vi "get response.vi"(8 "error in (no error)":errorcluster, 9 "time out (ms)":u32=30000, 10 "end char":string="^", 11 "port number":refnum<visa-resource-name>) -> (0 "error out":errorcluster, 1 "timed out":bool, 2 "response":string, 3 "port number out":refnum<visa-resource-name>)   [LabVIEW 2012]
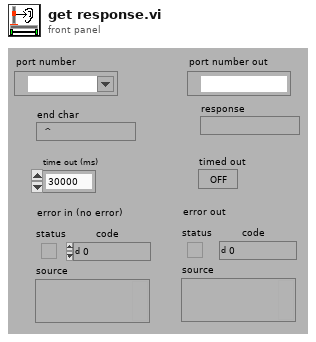
[diagram p1: front panel]
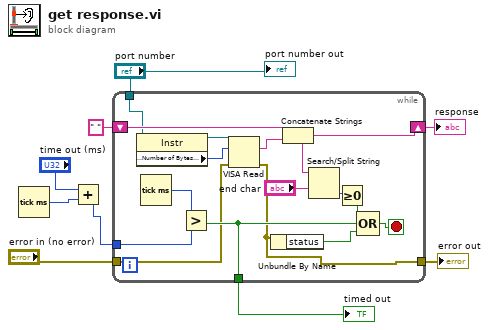
[diagram p0: block diagram]
diagram:
  n1 = Tick Count (ms)() -> (millisecond timer value=w3:u32)
  n2 = Add(x="time out (ms)", y=w3) -> (x+y=w2:u32)
  n3 = while {
    tunnel: [w17] -> w1
    tunnel: w2 -> [w19]
    tunnel: [w11] -> w7
    tunnel: "error in (no error)" -> [w13]
    shift-left: " " -> [w25]
    shift-right: [w24] -> w6
    tunnel: "port number" -> [w16]
    stop <- w22 stop-if-true
    n4 = property class="Instr"(reference=w16) -> (reference out=w15:refnum<visa-resource-name>, "Serial Settings:Number of Bytes at Serial Port"=w12:u32)  [unwired: 1 in, 1 out]
    n5 = Tick Count (ms)() -> (millisecond timer value=w20:u32)
    n6 = Greater?(x=w20, y=w19) -> (0:w17:bool)
    n7 = VISA Read(VISA resource name=w15, byte count=w12, error in (no error)=w13) -> (read buffer=w14:string, error out=w11:errorcluster)  [unwired: 2 out]
    n8 = Unbundle By Name(w11) -> ("status"=w10:bool)
    n9 = Concatenate Strings(w25, w14) -> (w24:string)
    n10 = Search/Split String(string=w24, search string/char (-)="end char") -> (offset of match=w23:i32)  [unwired: 1 in, 2 out]
    n11 = Greater Or Equal To 0?(x=w23) -> (x >= 0?=w18:bool)
    n12 = Compound Arithmetic op=OR(w18, w17, w10) -> (w22:bool)
  }
  "error out" <- w7
  "response" <- w6
  "timed out" <- w1
  "port number out" <- "port number"
